vi "libssh2_knownhost_readfile - invalid known hosts collection - returns zero.vi"() -> ()   [LabVIEW 2013, in "libssh2_tests.lvlib"]
uses:
  libssh2_tests.lvlib
  libssh2/Host Key Database Refnum.ctl
  libssh2/libssh2_init_default.vi
  <vilib>/addons/_JKI Toolkits/Caraya/classes/Assert/Assert Equal Value_Variant.vi
  <vilib>/addons/_JKI Toolkits/Caraya/classes/Test/Test.lvclass
  libssh2/libssh2.lvlib
  <vilib>/addons/_JKI Toolkits/Caraya/classes/Assert/Assert.lvclass
panel:
  out "error out":errorcluster
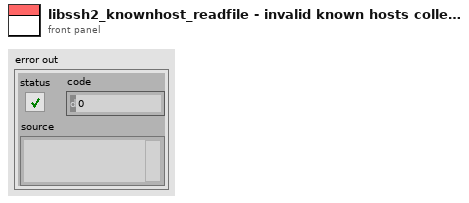
[diagram p1: front panel]
types:
  T1 = typedef "libssh2.lvlib/Session Refnum.ctl" = refnum<k1>
  T2 = typedef "libssh2.lvlib/Host Key Database Refnum.ctl" = refnum<k1>
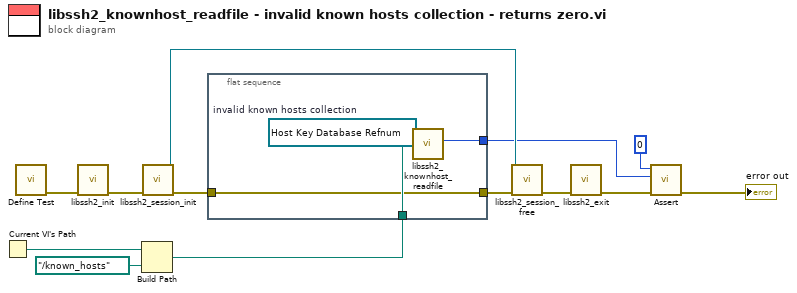
[diagram p0: block diagram]
diagram:
  n1 = Current VI's Path() -> (path=w5:path)
  n2 = call <vilib>:"Define Test.vi"() -> ("error out"=w12:errorcluster)  [unwired: 10 in, 1 out]
  n3 = call-poly "libssh2_init.vi"("error in (no error)"=w12) -> ("error out"=w11:errorcluster)  [unwired: 10 in]
  n4 = Build Path(base path=w5, name or relative path=path "../known_hosts" ("filename")) -> (appended path=w3:path)
  n5 = call "libssh2_session_init.vi"("error in (no error)"=w11) -> ("error out"=w2:errorcluster, "session"=w8:T1)  [unwired: 9 in]
  n6 = flat-sequence {
    tunnel: [w17] -> w7
    tunnel: w3 -> [w15]
    tunnel: w2 -> [w14]
    tunnel: [w14] -> w1
    frame #0 {
      w16 = T2 refnum items=["known host database"]  # invalid known hosts collection
      n7 = call "libssh2_knownhost_readfile.vi"("filename"=w15, "known hosts collection"=w16) -> ("hosts added"=w17:i32)  [unwired: 8 in, 1 out]
    }
  }
  n8 = call "libssh2_session_free.vi"("error in (no error)"=w1, "session"=w8) -> ("error out"=w10:errorcluster)  [unwired: 9 in]
  n9 = call "libssh2_exit.vi"("error in (no error)"=w10) -> ("error out"=w9:errorcluster)  [unwired: 10 in]
  n10 = call-poly <vilib>:"Assert.vi"("error in (no error)"=w9, "Y"=w7, "X"=0 ("hosts added")) -> ("error out"=→"error out":errorcluster)  [unwired: 7 in, 1 out]
